vi "Spin Coar ReadStops(SubVI).vi"(0 "VISA Refnum in":refnum<visa-resource-name>, 5 "stop":bool, 9 "bytes to read":u32) -> (1 "error out":errorcluster, 2 "Boolean":bool, 3 "Match Number":i32, 4 "Match 1":u8, 6 "Match 2":u8, 8 "Match 3":u8, 10 "Match 4":u8, 11 "read string":string, 12 "String After Match":string, 13 "String Match":string, 14 "String Before Match":string, 15 "Match 5":u8)   [LabVIEW 2018]
uses:
  <vilib>/Instr/_visa.llb/VISA Configure Serial Port (Instr).vi
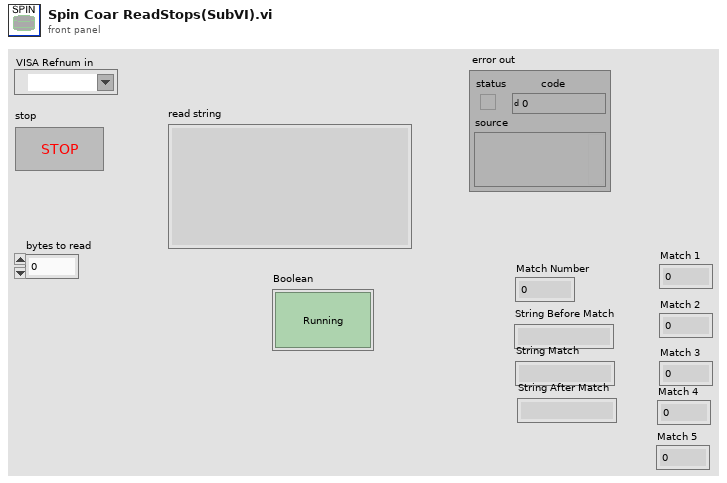
[diagram p1: front panel]
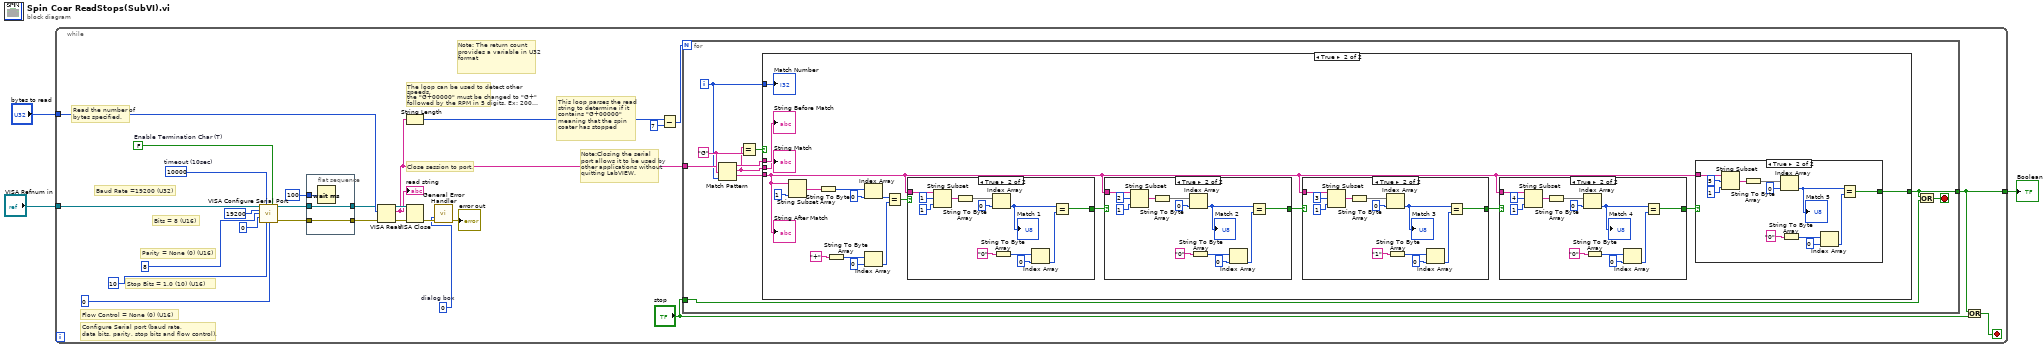
[diagram p0: block diagram]
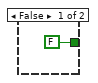
[diagram p2: hidden frame]
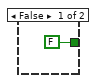
[diagram p3: hidden frame]
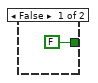
[diagram p4: hidden frame]
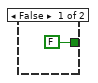
[diagram p5: hidden frame]
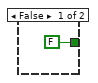
[diagram p6: hidden frame]
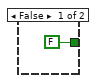
[diagram p7: hidden frame]
diagram:
  n1 = while {
    tunnel: "VISA Refnum in" -> [w21]
    tunnel: "bytes to read" -> [w20]
    tunnel: [w13] -> w1
    stop <- w4 stop-if-true
    w5 = 0  # dialog box
    w27 = FALSE  # Enable Termination Char (T)
    w28 = u32 10000  # timeout (10sec)
    # "Note: The return count provides a variable in U32 format"
    # "The loop can be used to detect other speeds,\nthe \"G+00000\" must be changed to \"G+\" \nfollowed by the RPM in 5 digits. Ex: 200 RPM\nwould be designated by \"G+00200\""
    # "This loop parses the read string to determine if it contains \"G+00000\" meaning that the spin coater has stopped"
    # "Flow Control = None (0) (U16)"
    # "Stop Bits = 1.0 (10) (U16)"
    # "Baud Rate =19200 (U32)"
    # "Bits = 8 (U16)"
    # "Parity = None (0) (U16)"
    # "Read the number of bytes specified."
    # "Note:Closing the serial port allows it to be used by other applications without\nquitting LabVIEW."
    # "Configure Serial port (baud rate,\ndata bits, parity, stop bits and flow control)."
    # "Close session to port."
    n2 = call-poly "VISA Configure Serial Port"("VISA resource name"=w21, "timeout (10sec)"=w28, "Enable Termination\nChar (T)"=w27, "baud rate (9600)"=u32 19200, "data bits (8)"=u16 8, "parity (0:none)"=u32 0, "stop bits (10: 1 bit)"=u16 10, "flow control (0:none)"=u16 0) -> ("VISA resource name out"=w9:refnum<visa-resource-name>, "error out"=w7:errorcluster)  [unwired: 6 in]
    n3 = flat-sequence {
      tunnel: u32 100 -> [w32]
      tunnel: [w31] -> w10
      tunnel: w9 -> [w31]
      tunnel: [w30] -> w8
      tunnel: w7 -> [w30]
      frame #0 {
        n4 = Wait (ms)(milliseconds to wait=w32) -> ()  [unwired: 1 out]
      }
    }
    n5 = VISA Read(VISA resource name=w10, byte count=w20, error in (no error)=w8) -> (VISA resource name out=w26:refnum<visa-resource-name>, read buffer=w12:string, error out=w6:errorcluster)  [unwired: 1 out]
    "read string" <- w12
    n6 = String Length(string=w12) -> (length=w16:i32)
    n7 = VISA Close(VISA resource name=w26, error in (no error)=w6) -> (error out=w29:errorcluster)
    n8 = call <vilib>:"General Error Handler.vi"("type of dialog (OK msg:1)"=w5, "error in (no error)"=w29) -> ("error out"=→"error out":errorcluster)  [unwired: 9 in, 4 out]
    n9 = Subtract(x=w16, y=u32 7) -> (x-y=w17:u32)
    n10 = for {
      N: w17 -> [_]
      tunnel: w12 -> [w41]
      tunnel: [w33] -> w13
      tunnel: "stop" -> [w34]
      i -> [w37]
      stop <- w35 stop-if-true
      w42 = "G"
      n11 = Match Pattern(string=w41, regular expression=w42, offset (0)=w37) -> (before substring=w40:string, match substring=w39:string, after substring=w38:string)  [unwired: 1 out]
      n12 = Equal?(x=w39, y=w42) -> (x = y?=w36:bool)
      n13 = case shown="True" w36 {
        tunnel: w40 -> [_ w62]
        tunnel: w39 -> [_ w61]
        tunnel: w38 -> [_ w46]
        tunnel: w37 -> [_ w60]
        tunnel: [FALSE w44] -> w33
        frame False {
        }
        frame True {
          n14 = String Subset(string=w46, length (rest)=1) -> (substring=w58:string)  [unwired: 1 in]
          n15 = String To Byte Array(string=w58) -> (unsigned byte array=w52:u8[])
          n16 = String To Byte Array(string="+") -> (unsigned byte array=w57:u8[])
          n17 = Index Array(array=w52, index=0) -> (element=w51:u8)
          n18 = Index Array(array=w57, index=0) -> (element=w55:u8)
          n19 = Equal?(x=w51, y=w55) -> (x = y?=w50:bool)
          n20 = case shown="True" w50 {
            tunnel: [FALSE w124] -> w49
            tunnel: w46 -> [_ w116]
            frame False {
            }
            frame True {
              n21 = String Subset(string=w116, offset (0)=1, length (rest)=1) -> (substring=w119:string)
              n22 = String To Byte Array(string=w119) -> (unsigned byte array=w118:u8[])
              n23 = Index Array(array=w118, index=0) -> (element=w122:u8)
              "Match 1" <- w122
              n24 = String To Byte Array(string="0") -> (unsigned byte array=w126:u8[])
              n25 = Index Array(array=w126, index=0) -> (element=w123:u8)
              n26 = Equal?(x=w122, y=w123) -> (x = y?=w124:bool)
            }
          }
          n27 = case shown="True" w49 {
            tunnel: [FALSE w111] -> w48
            tunnel: w46 -> [_ w104]
            frame False {
            }
            frame True {
              n28 = String Subset(string=w104, offset (0)=2, length (rest)=1) -> (substring=w106:string)
              n29 = String To Byte Array(string=w106) -> (unsigned byte array=w105:u8[])
              n30 = Index Array(array=w105, index=0) -> (element=w109:u8)
              "Match 2" <- w109
              n31 = String To Byte Array(string="0") -> (unsigned byte array=w113:u8[])
              n32 = Index Array(array=w113, index=0) -> (element=w110:u8)
              n33 = Equal?(x=w109, y=w110) -> (x = y?=w111:bool)
            }
          }
          n34 = case shown="True" w48 {
            tunnel: [FALSE w98] -> w47
            tunnel: w46 -> [_ w91]
            frame False {
            }
            frame True {
              n35 = String Subset(string=w91, offset (0)=3, length (rest)=1) -> (substring=w93:string)
              n36 = String To Byte Array(string=w93) -> (unsigned byte array=w92:u8[])
              n37 = Index Array(array=w92, index=0) -> (element=w96:u8)
              "Match 3" <- w96
              n38 = String To Byte Array(string="1") -> (unsigned byte array=w100:u8[])
              n39 = Index Array(array=w100, index=0) -> (element=w97:u8)
              n40 = Equal?(x=w96, y=w97) -> (x = y?=w98:bool)
            }
          }
          n41 = case shown="True" w47 {
            tunnel: [FALSE w85] -> w45
            tunnel: w46 -> [_ w78]
            frame False {
            }
            frame True {
              n42 = String Subset(string=w78, offset (0)=4, length (rest)=1) -> (substring=w80:string)
              n43 = String To Byte Array(string=w80) -> (unsigned byte array=w79:u8[])
              n44 = Index Array(array=w79, index=0) -> (element=w83:u8)
              "Match 4" <- w83
              n45 = String To Byte Array(string="0") -> (unsigned byte array=w87:u8[])
              n46 = Index Array(array=w87, index=0) -> (element=w84:u8)
              n47 = Equal?(x=w83, y=w84) -> (x = y?=w85:bool)
            }
          }
          n48 = case shown="True" w45 {
            tunnel: [FALSE w72] -> w44
            tunnel: w46 -> [_ w65]
            frame False {
            }
            frame True {
              n49 = String Subset(string=w65, offset (0)=5, length (rest)=1) -> (substring=w67:string)
              n50 = String To Byte Array(string=w67) -> (unsigned byte array=w66:u8[])
              n51 = Index Array(array=w66, index=0) -> (element=w70:u8)
              "Match 5" <- w70
              n52 = String To Byte Array(string="0") -> (unsigned byte array=w74:u8[])
              n53 = Index Array(array=w74, index=0) -> (element=w71:u8)
              n54 = Equal?(x=w70, y=w71) -> (x = y?=w72:bool)
            }
          }
          "String Before Match" <- w62
          "String Match" <- w61
          "String After Match" <- w46
          "Match Number" <- w60
        }
      }
      n55 = Or(x=w33, y=w34) -> (x .or. y?=w35:bool)
    }
    n56 = Or(x=w13, y="stop") -> (x .or. y?=w4:bool)
  }
  "Boolean" <- w1
